vi "mWmotor_move_to absolute.vi"(8 "error in (no error)":errorcluster, 9 "absolute possition(rev)":dbl, 10 "milliseconds to wait":u32=100, 11 "MW motor":refnum<visa-resource-name>) -> (0 "error out":errorcluster, 3 "VISA resource name out":refnum<visa-resource-name>)   [LabVIEW 2019]
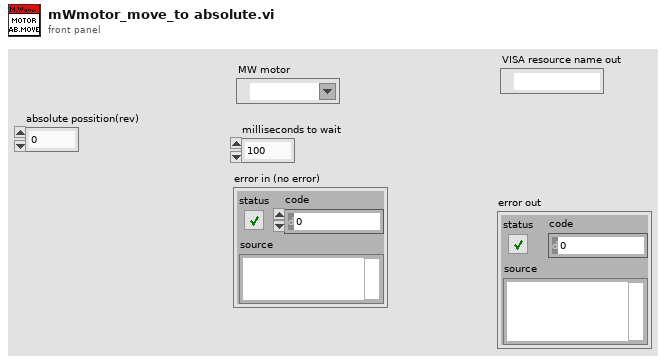
[diagram p1: front panel]
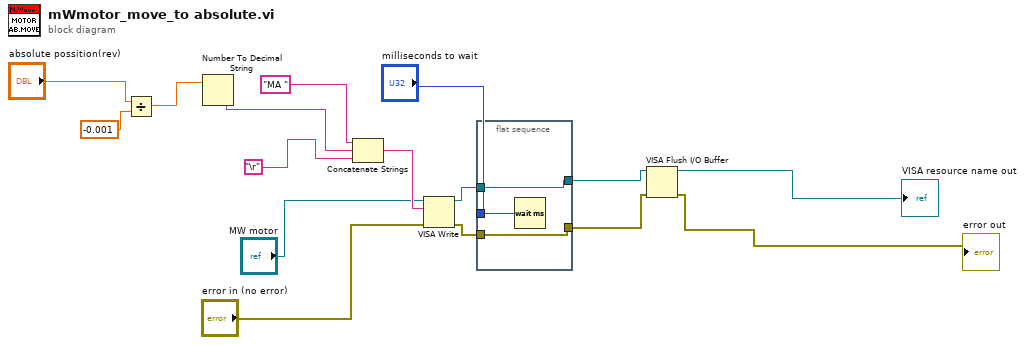
[diagram p0: block diagram]
diagram:
  n1 = Divide(x="absolute possition(rev)", y=-0.001) -> (x/y=w8:dbl)
  n2 = Number To Decimal String(number=w8) -> (decimal integer string=w6:string)  [unwired: 1 in]
  n3 = Concatenate Strings("MA " ("string"), w6, "\r") -> (w16:string)
  n4 = VISA Write(VISA resource name="MW motor", write buffer=w16, error in (no error)="error in (no error)") -> (VISA resource name out=w12:refnum<visa-resource-name>, error out=w13:errorcluster)  [unwired: 1 out]
  n5 = flat-sequence {
    tunnel: [w19] -> w3
    tunnel: w13 -> [w19]
    tunnel: [w18] -> w2
    tunnel: w12 -> [w18]
    tunnel: "milliseconds to wait" -> [w17]
    frame #0 {
      n6 = Wait (ms)(milliseconds to wait=w17) -> ()  [unwired: 1 out]
    }
  }
  n7 = VISA Flush I/O Buffer(VISA resource name=w2, error in (no error)=w3) -> (VISA resource name out=→"VISA resource name out":refnum<visa-resource-name>, error out=→"error out":errorcluster)  [unwired: 1 in]
